vi "Do.vi"(7 "Topic Actor in":refnum<class "Topic Actor.lvclass">, 8 "error in (no error)":errorcluster, 11 "Topic Actor Command in":refnum<class "Topic Actor Unsubscribe Command.lvclass">) -> (0 "error out":errorcluster, 3 "Topic Actor Command out":refnum<class "Topic Actor Unsubscribe Command.lvclass">, 5 "Topic Actor out":refnum<class "Topic Actor.lvclass">)   [LabVIEW 2016, in "Stream Mediator.lvlib" / "Topic Actor Unsubscribe Command.lvclass"]
doc: "--\nCopyright © 2017 Composed SystemsI All rights reserved.\n\nAuthor: Jon McBee <jon.mcbee@composed.io>\n\nThis library is provided \"AS IS\" ,WITHOUT WARRANTIES OR\nCONDITIONS OF ANY KIND, either express or implied.\n\nComposed Systems -- composed.io\n\nStream 0.0.1.1\nJon McBee - Composed Systems\nCopyright (c) 2017, Composed Systems"
uses:
  <userlib>/Composed Systems/Stream/Mediator/Classes/Topic Actor Unsubscribe Command/Topic Actor Unsubscribe Command.lvclass
  <userlib>/Composed Systems/Stream/Mediator/Classes/Topic Actor/Topic Actor.lvclass
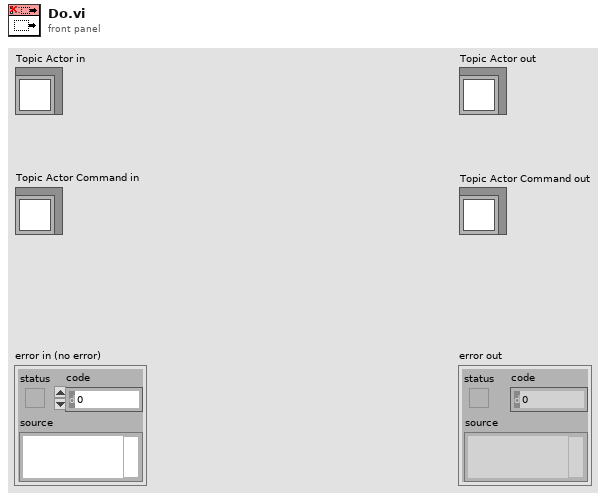
[diagram p1: front panel]
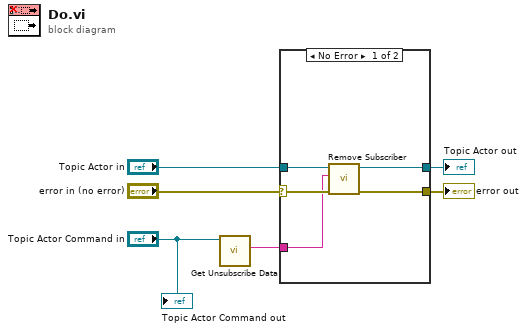
[diagram p0: block diagram]
diagram:
  n1 = call <userlib>:"Get Unsubscribe Data.vi"("Topic Actor Unsubscribe Command in"="Topic Actor Command in") -> ("Subscriber Name"=w1:string)  [unwired: 8 in, 2 out]
  n2 = case shown="No Error" "error in (no error)" {
    selector: "error in (no error)" -> [w9 w12]
    tunnel: [w8 w12] -> w4
    tunnel: "Topic Actor in" -> [w11 w13]
    tunnel: [w10 w13] -> w2
    tunnel: w1 -> [w7 _]
    frame No Error {
      n3 = call <userlib>:"Remove Subscriber.vi"("error in (no error)"=w9, "Topic Name"=w7, "Topic Actor in"=w11) -> ("error out"=w8:errorcluster, "Topic Actor out"=w10:refnum<class "Topic Actor.lvclass">)  [unwired: 7 in]
    }
    frame Error {
    }
  }
  "error out" <- w4
  "Topic Actor out" <- w2
  "Topic Actor Command out" <- "Topic Actor Command in"
